vi "PID Control.vi"() -> ()   [LabVIEW 2014]
uses:
  <vilib>/rvi/Emulation/niFpgaGetClockAttributes.vi
  <vilib>/rvi/Emulation/niFpgaSctlEmulationGetInTimedLoop.vi
  <vilib>/rvi/Emulation/niFpgaEmulationReportErrorSimple.vi
  <vilib>/rvi/Emulation/niFpgaCriticalErrorInLSC.vi
  <vilib>/addons/control/pid/fpga.llb/XNode/niFpgaPID.xnode
panel:
  in  "FPGA Count(uSec)":u32
  out "FPGA PID Output":fxp<+/-,16,16>
  out "Latency":u8
  in  "FPGA SP":fxp<+/-,16,16>=700.0
  in  "FPGA PID reset?":bool
  in  "output range":T1={"output high"=32767.0, "output low"=-32768.0}
  in  "PID gains":T2={"proportional gain (Kc)"=1.0, "integral gain (Kc*Ts/Ti)"=1.66796875, "derivative gain (Kc*Td/Ts)"=0.0}
  in  "FPGA PV":fxp<+/-,16,16>
  in  "Loop Time(uSec)":u32
  in  "FPGA Stop":bool
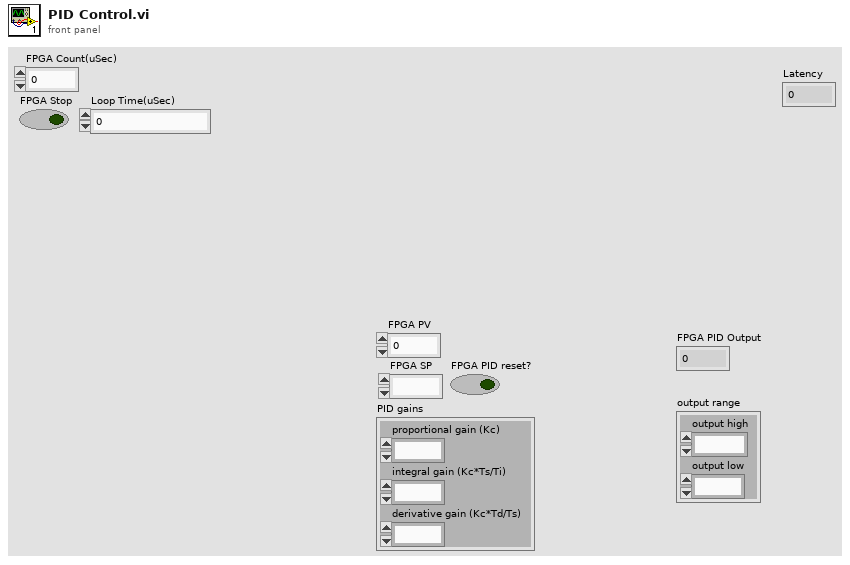
[diagram p1: front panel]
types:
  T1 = cluster{"output high":fxp<+/-,16,16>, "output low":fxp<+/-,16,16>}
  T2 = cluster{"proportional gain (Kc)":fxp<+/-,16,8>, "integral gain (Kc*Ts/Ti)":fxp<+/-,16,8>, "derivative gain (Kc*Td/Ts)":fxp<+/-,16,8>}
  T3 = cluster{"proportional gain (Kc)":i16, "integral gain (Kc*Ts/Ti)":i16, "derivative gain (Kc*Td/Ts)":i16}
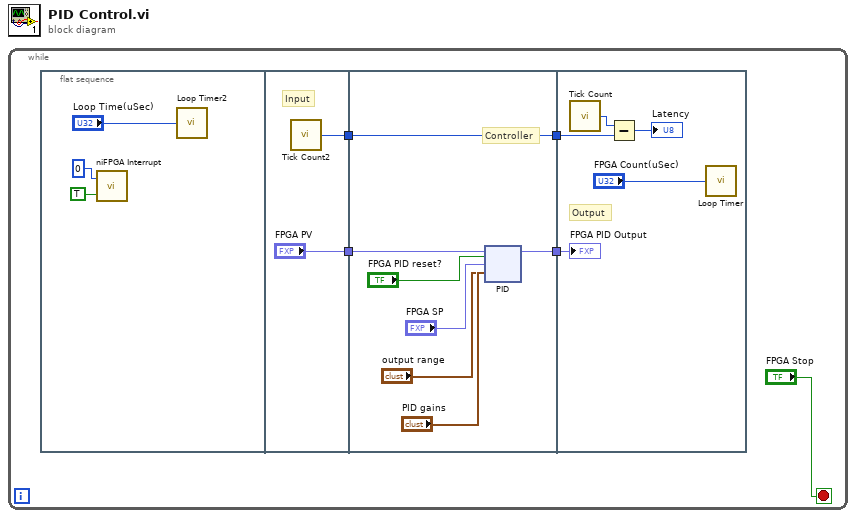
[diagram p0: block diagram]
diagram:
  n1 = while {
    stop <- "FPGA Stop" stop-if-true
    n2 = flat-sequence {
      tunnel: ["FPGA PV"] -> w3
      tunnel: [w10] -> w1
      tunnel: [w14] -> w4
      tunnel: w3 -> [w13]
      tunnel: [w11] -> w2
      tunnel: w1 -> [w11]
      tunnel: w4 -> [w49]
      tunnel: w2 -> [w47]
      frame #0 {
        n3 = call <vilib>:"niFPGA Interrupt.vi"("Wait Until Cleared (F)"=TRUE, "IRQ Number (0)"=u8 0) -> ()  [unwired: 1 in]
        n4 = call "Loop Timer2"("Count(uSec)"="Loop Time(uSec)") -> ()  [unwired: 1 out]
      }
      frame #1 {
        # "Input"
        n5 = call "Tick Count2"() -> ("Tick Count(Ticks)"=w10:u8)
      }
      frame #2 {
        # "Controller"
        n6 = xnode "PID"("process variable"=w13, "reset?"="FPGA PID reset?", "setpoint"="FPGA SP", "PID gains"="PID gains", "output range"="output range") -> ("output"=w14:fxp<+/-,16,16>)
      }
      frame #3 {
        # "Output"
        n7 = call "Tick Count"() -> ("Tick Count(Ticks)"=w48:u8)
        n8 = Subtract(x=w48, y=w47) -> (x-y=→"Latency":u8)
        n9 = call "Loop Timer"("Count(uSec)"="FPGA Count(uSec)") -> ()  [unwired: 1 out]
        "FPGA PID Output" <- w49
      }
    }
  }
